vi "DWORD2FLOAT.vi"(10 "Low":u16, 11 "High":u16) -> (3 "Float":sgl)   [LabVIEW 2018, in "SubVi.lvlib"]
uses:
  SubVi.lvlib
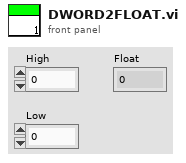
[diagram p1: front panel]
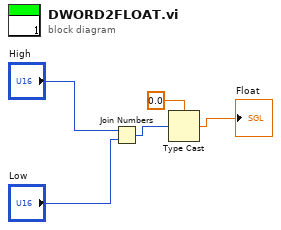
[diagram p0: block diagram]
diagram:
  n1 = Join Numbers(hi="High", lo="Low") -> ((hi.lo)=w2:u32)
  n2 = Type Cast(type=sgl 0.0, x=w2) -> (*(type *) &x=→"Float":sgl)
